vi "PV Software HEX String to U8.vi"(8 "error in (no error)":errorcluster, 11 "HEX Data (String)":string[](array[string])) -> (0 "error out":errorcluster, 3 "HEX Data (U16)":u8[][](array[numeric]) format="%x")   [LabVIEW 2023]
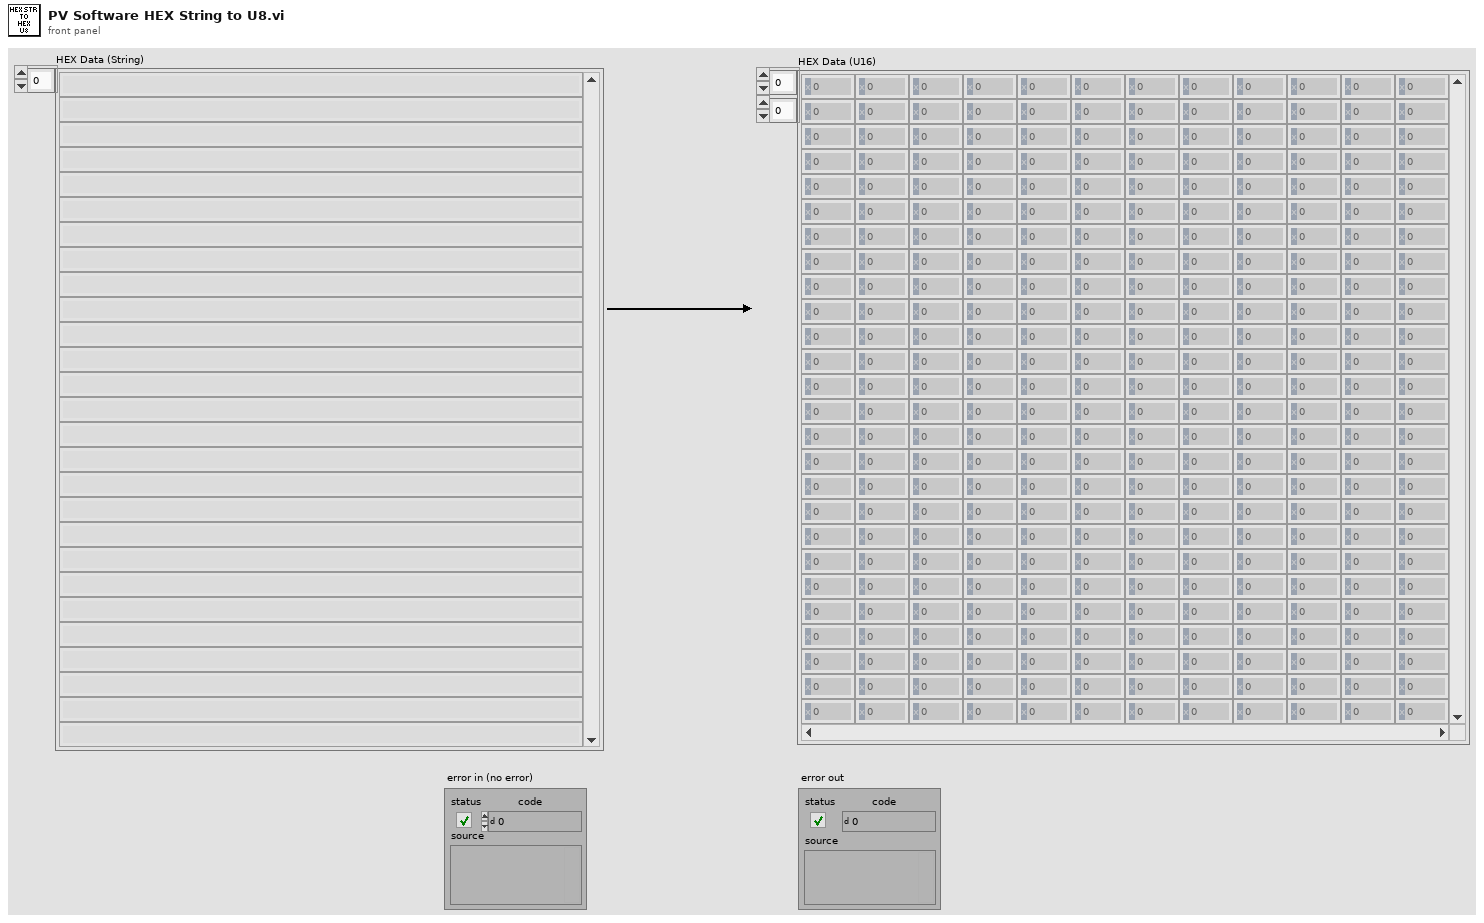
[diagram p1: front panel]
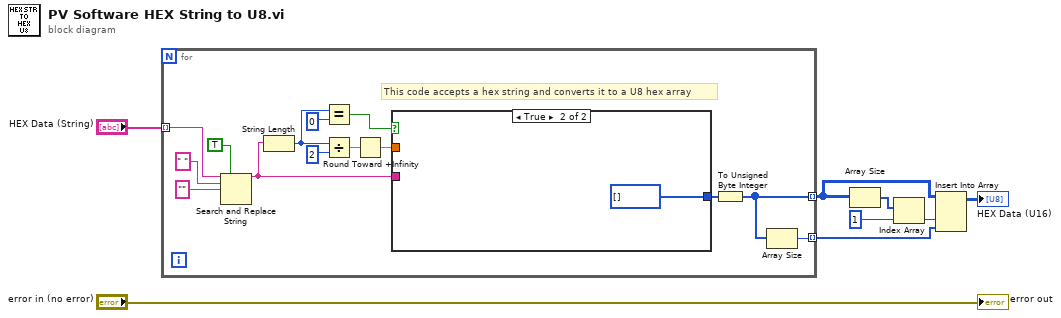
[diagram p0: block diagram]
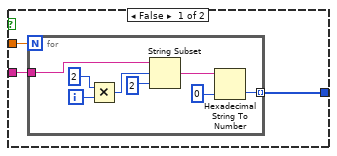
[diagram p2: hidden frame]
diagram:
  n1 = for {
    tunnel: "HEX Data (String)" -> [w12] mode=indexing
    tunnel: [w9] -> w4 mode=indexing
    tunnel: [w11] -> w6 mode=indexing
    # "This code accepts a hex string and converts it to a U8 hex array"
    n2 = Search and Replace String(replace all?=TRUE ("replace all? (F)"), input string=w12, search string=" ", replace string="" ("replace string (\"\")")) -> (result string=w15:string)  [unwired: 4 in, 3 out]
    n3 = String Length(string=w15) -> (length=w19:i32)
    n4 = Equal?(x=w19, y=0) -> (x = y?=w17:bool)
    n5 = Divide(x=w19, y=2) -> (x/y=w22:dbl)
    n6 = Round Toward +Infinity(x=w22) -> (ceil(x): smallest int >= x=w21:dbl)
    n7 = case shown="True" w17 {
      tunnel: w15 -> [w25 _]
      tunnel: w21 -> [w24 _]
      tunnel: [w23 u16[] []] -> w10
      frame False {
        n8 = for {
          N: w24 -> [_]
          tunnel: w25 -> [w31]
          tunnel: [w26] -> w23 mode=indexing
          i -> [w33]
          n9 = Multiply(x=2, y=w33) -> (x*y=w30:i32)
          n10 = String Subset(string=w31, offset (0)=w30, length (rest)=2 ("length (rest)")) -> (substring=w27:string)
          n11 = Hexadecimal String To Number(string=w27, default (0uL)=u16 0 ("default (0 U32)")) -> (number=w26:u16)  [unwired: 1 in, 1 out]
        }
      }
      frame True {
      }
    }
    n12 = To Unsigned Byte Integer(number=w10) -> (unsigned 8bit integer=w9:u8[])
    n13 = Array Size(array=w9) -> (size(s)=w11:i32)
  }
  n14 = Array Size(array=w4) -> (size(s)=w3:i32[])
  n15 = Index Array(array=w3, index=u8 1) -> (element=w1:i32)
  n16 = Insert Into Array(array=w4, index (col)=w1, new element=w6) -> (→"HEX Data (U16)":u8[][])  [unwired: 1 in]
  "error out" <- "error in (no error)"
